vi "9219_Class_to_Data.vi"(8 "error in (no error)":errorcluster, 11 "9219 in":refnum<class "9219.lvclass">) -> (0 "error out":errorcluster, 2 "9219 Config":T1 {"Conversion Time" items=["High Speed", "Best 60 Hz Rejection", "Best 50 Hz Rejection", "High Resolution"]; "TCoupleType" items=["J", "K", "T", "E", "R", "S", "N", "B"]; "DegreeRange" items=["Raw units", "Degrees Kelvin", "Degrees Celsius", "Degrees Fahrenheit", "Degrees Rankine"]; "RtdType" items=["TCR3851"=1, "TCR3750"=2, "TCR3916"=3, "TCR3920"=4, "TCR3911"=5, "TCR3928"=6, "Custom"=0]}, 3 "9219 out":refnum<class "9219.lvclass">)   [LabVIEW 2019, in "Modules.lvlib" / "9219.lvclass"]
uses:
  9219.lvclass
  9219 Config.ctl
  9219.lvclass/9219.ctl
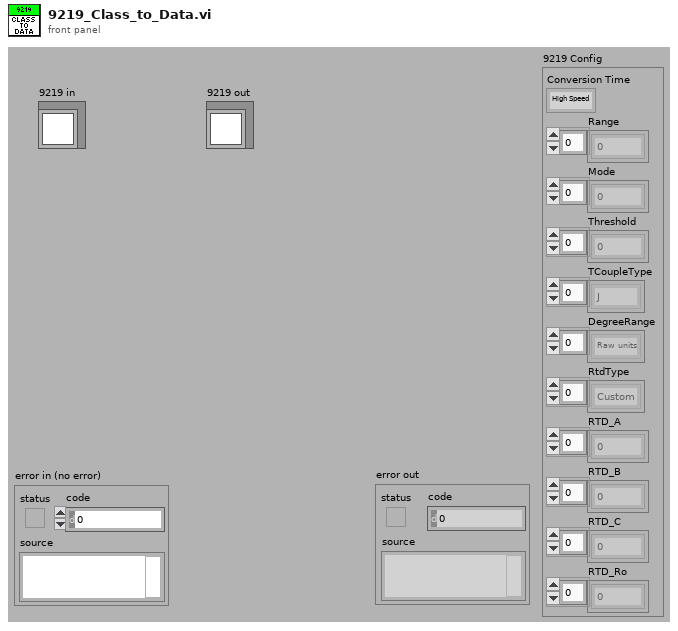
[diagram p1: front panel]
types:
  T1 = typedef "Modules.lvlib/9219.lvclass/9219 Config.ctl" = cluster{"Conversion Time":u16, "Range":u8[], "Mode":u8[], "Threshold":dbl[], "TCoupleType":u8[], "DegreeRange":u8[], "RtdType":u8[], "RTD_A":dbl[], "RTD_B":dbl[], "RTD_C":dbl[], "RTD_Ro":dbl[]}
  T2 = cluster{"Degree range":u32, "Digital threshold":dbl, "Range / Mode":u32, "RTD type":u32, "RTD A":dbl, "RTD B":dbl, "RTD C":dbl, "RTD Ro":dbl, "Thermocouple type":u32}[]
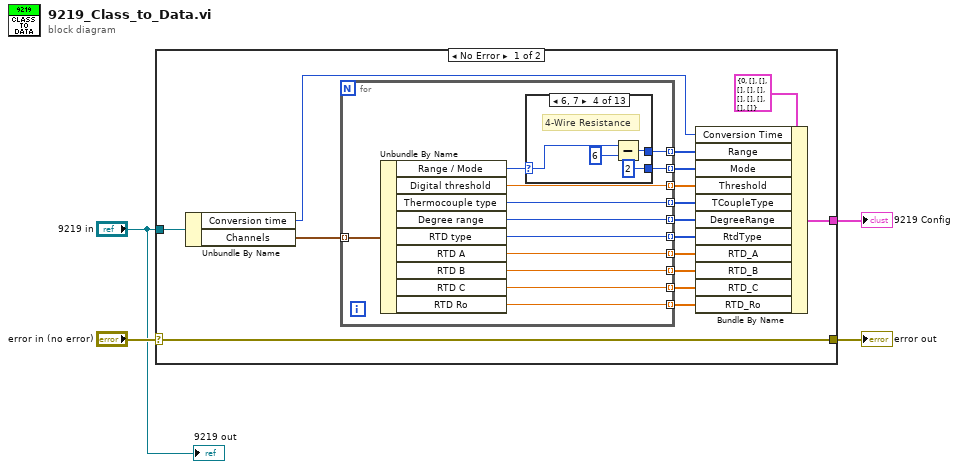
[diagram p0: block diagram]
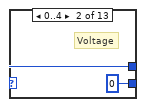
[diagram p3: hidden frame]
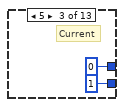
[diagram p4: hidden frame]
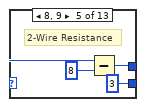
[diagram p5: hidden frame]
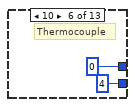
[diagram p6: hidden frame]
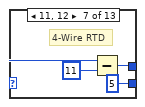
[diagram p7: hidden frame]
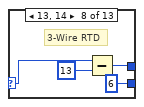
[diagram p8: hidden frame]
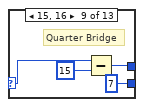
[diagram p9: hidden frame]
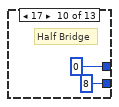
[diagram p10: hidden frame]
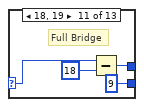
[diagram p11: hidden frame]
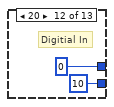
[diagram p12: hidden frame]
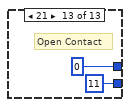
[diagram p13: hidden frame]
diagram:
  n1 = case shown="No Error" "error in (no error)" {
    selector: "error in (no error)" -> [w16 w69]
    tunnel: [w16 w69] -> w3
    tunnel: "9219 in" -> [w20 _]
    tunnel: [w7 _] -> w2
    frame No Error {
      n2 = Unbundle By Name(w20) -> ("Conversion time"=w17:u32, "Channels"=w19:T2)
      n3 = for {
        tunnel: w19 -> [w32] mode=indexing
        tunnel: [w31] -> w15 mode=indexing
        tunnel: [w30] -> w14 mode=indexing
        tunnel: [w29] -> w13 mode=indexing
        tunnel: [w28] -> w12 mode=indexing
        tunnel: [w27] -> w11 mode=indexing
        tunnel: [w26] -> w10 mode=indexing
        tunnel: [w21] -> w9 mode=indexing
        tunnel: [w25] -> w8 mode=indexing
        tunnel: [w23] -> w6 mode=indexing
        tunnel: [w22] -> w5 mode=indexing
        n4 = Unbundle By Name(w32) -> ("Range / Mode"=w24:u32, "Digital threshold"=w25:dbl, "Thermocouple type"=w21:u32, "Degree range"=w26:u32, "RTD type"=w27:u32, "RTD A"=w28:dbl, "RTD B"=w29:dbl, "RTD C"=w30:dbl, "RTD Ro"=w31:dbl)
        n5 = case shown="6, 7" w24 {
          selector: w24 -> [_ w33 _ w39 w43 _ w49 w53 w57 _ w63 _ _]
          tunnel: [_ w33 u32 0 ("Range / Mode") w37 w41 u32 0 ("Range / Mode") w47 w51 w55 u32 0 ("Range / Mode") w61 u32 0 ("Range / Mode") u32 0 ("Range / Mode")] -> w23
          tunnel: [_ u8 0 ("Numeric") u8 1 ("Numeric") u8 2 ("Numeric") u8 3 ("Numeric") u8 4 ("Numeric") u8 5 ("Numeric") u8 6 ("Numeric") u8 7 ("Numeric") u8 8 ("Numeric") u8 9 ("Numeric") u8 10 ("Numeric") u8 11 ("Numeric")] -> w22
          frame Default {
          }
          frame 0..4 {
            # "Voltage"
          }
          frame 5 {
            # "Current"
          }
          frame 6, 7 {
            # "4-Wire Resistance"
            n6 = Subtract(x=w39, y=u32 6) -> (x-y=w37:u32)
          }
          frame 8, 9 {
            # "2-Wire Resistance"
            n7 = Subtract(x=w43, y=u32 8) -> (x-y=w41:u32)
          }
          frame 10 {
            # "Thermocouple"
          }
          frame 11, 12 {
            # "4-Wire RTD"
            n8 = Subtract(x=w49, y=u32 11) -> (x-y=w47:u32)
          }
          frame 13, 14 {
            # "3-Wire RTD"
            n9 = Subtract(x=w53, y=u32 13) -> (x-y=w51:u32)
          }
          frame 15, 16 {
            # "Quarter Bridge"
            n10 = Subtract(x=w57, y=u32 15) -> (x-y=w55:u32)
          }
          frame 17 {
            # "Half Bridge"
          }
          frame 18, 19 {
            # "Full Bridge"
            n11 = Subtract(x=w63, y=u32 18) -> (x-y=w61:u32)
          }
          frame 20 {
            # "Digitial In"
          }
          frame 21 {
            # "Open Contact"
          }
        }
      }
      n12 = Bundle By Name(cluster=T1 {"Conversion Time"=0, "Range"=[], "Mode"=[], "Threshold"=[], "TCoupleType"=[], "DegreeRange"=[], "RtdType"=[], "RTD_A"=[], "RTD_B"=[], "RTD_C"=[], "RTD_Ro"=[]} ("9219 Config"), "Conversion Time"=w17, "Range"=w6, "Mode"=w5, "Threshold"=w8, "TCoupleType"=w9, "DegreeRange"=w10, "RtdType"=w11, "RTD_A"=w12, "RTD_B"=w13, "RTD_C"=w14, "RTD_Ro"=w15) -> (w7:T1)
    }
    frame Error {
    }
  }
  "error out" <- w3
  "9219 Config" <- w2
  "9219 out" <- "9219 in"
